vi "Register gRPC Methods.vi"(8 "error in (no error)":errorcluster, 11 "Template Server in":refnum<class "TempController_server.lvclass">) -> (0 "error out":errorcluster, 3 "Template Server out":refnum<class "TempController_server.lvclass">)   [LabVIEW 2019, in "TempController_server.lvlib" / "TempController_server.lvclass"]
uses:
  TempController_server.lvclass
  typeDefs/Server Internal UEs.ctl
  typeDefs/Server Internal Message.ctl
  typeDefs/Server gRPC UEs.ctl
  <vilib>/gRPC/LabVIEW gRPC Library/Server API/typeDefs/gRPCId Cluster.ctl
  <vilib>/gRPC/LabVIEW gRPC Library/Server API/typeDefs/grpcId.ctl
  TempController_server.lvclass/TempController_server.ctl
  <vilib>/gRPC/LabVIEW gRPC Library/gprc-lvsupport-release.lvlib
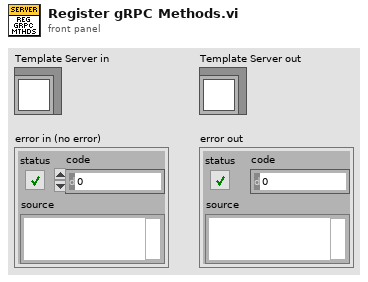
[diagram p1: front panel]
types:
  T1 = typedef "TempController_server.lvlib/TempController_server.lvclass/Server gRPC UEs.ctl" = cluster{"TemperatureControllerService_Measure gRPC UE":refnum<user-event>, "TemperatureControllerService_Configure gRPC UE":refnum<user-event>}
  T2 = typedef "TempController_server.lvlib/TempController_server.lvclass/Server Internal UEs.ctl" = cluster{"TemperatureControllerService_Measure Internal UE":refnum<user-event>, "TemperatureControllerService_Configure Internal UE":refnum<user-event>}
  T3 = typedef "gprc-lvsupport-release.lvlib/grpcId.ctl" = u64
  T4 = typedef "TempController_server.lvlib/TempController_server.lvclass/Server Internal Message UE.ctl" = refnum<user-event>
  T5 = typedef "gprc-lvsupport-release.lvlib/gRPCId Cluster UE.ctl" = refnum<user-event>
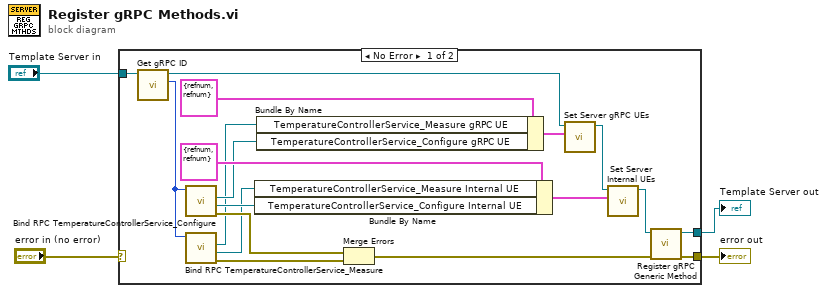
[diagram p0: block diagram]
diagram:
  n1 = case shown="No Error" "error in (no error)" {
    selector: "error in (no error)" -> [_ w23]
    tunnel: "Template Server in" -> [w21 w24]
    tunnel: [w14 w23] -> w3
    tunnel: [w12 w24] -> w2
    frame No Error {
      n2 = call "Get gRPC ID.vi"("OOP Server in"=w21) -> ("gRPC ID"=w11:T3, "OOP Server out"=w22:refnum<class "TempController_server.lvclass">)  [unwired: 9 in]
      n3 = call "Bind RPC TemperatureControllerService_Configure.vi"("gRPCid server in"=w11) -> ("error out"=w10:errorcluster, "TemperatureControllerService_Configure Internal UE"=w8:T4, "TemperatureControllerService_Configure gRPC UE"=w9:T5)  [unwired: 7 in, 1 out]
      n4 = call "Bind RPC TemperatureControllerService_Measure.vi"("gRPCid server in"=w11) -> ("error out"=w7:errorcluster, "TemperatureControllerService_Measure Internal UE"=w6:T4, "TemperatureControllerService_Measure gRPC UE"=w5:T5)  [unwired: 7 in, 1 out]
      n5 = Bundle By Name ("Bundle Internal UEs")(cluster=T2 {"TemperatureControllerService_Measure Internal UE"=refnum, "TemperatureControllerService_Configure Internal UE"=refnum} ("Server Internal UEs"), "TemperatureControllerService_Measure Internal UE"=w6, "TemperatureControllerService_Configure Internal UE"=w8) -> (w20:T2)
      n6 = Bundle By Name ("Bundle gRPC UEs")(cluster=T1 {"TemperatureControllerService_Measure gRPC UE"=refnum, "TemperatureControllerService_Configure gRPC UE"=refnum} ("gRPC Server Method Events"), "TemperatureControllerService_Measure gRPC UE"=w5, "TemperatureControllerService_Configure gRPC UE"=w9) -> (w17:T1)
      n7 = Merge Errors(w10, w7) -> (w15:errorcluster)
      n8 = call "Set Server gRPC UEs.vi"("Server RPC Methods"=w17, "OOP Server in"=w22) -> ("OOP Server out"=w18:refnum<class "TempController_server.lvclass">)  [unwired: 9 in]
      n9 = call "Set Server Internal UEs.vi"("Server Internal UEs"=w20, "OOP Server in"=w18) -> ("OOP Server out"=w13:refnum<class "TempController_server.lvclass">)  [unwired: 9 in]
      n10 = call "Register gRPC Generic Method.vi"("error in (no error)"=w15, "Template Server in"=w13) -> ("error out"=w14:errorcluster, "Template Server out"=w12:refnum<class "TempController_server.lvclass">)  [unwired: 8 in]
    }
    frame Error {
    }
  }
  "error out" <- w3
  "Template Server out" <- w2
